vi "Read Data.vi"(8 "error in (no error)":errorcluster caption="错误输入（无错误）", 11 "Primary Productivity 输入":refnum<class "Primary Productivity.lvclass">) -> (0 "error out":errorcluster caption="错误输出", 3 "Primary Productivity 输出":refnum<class "Primary Productivity.lvclass">)   [LabVIEW 2016, in "Primary Productivity.lvclass"]
uses:
  Primary Productivity.lvclass
  Primary Productivity.lvclass/Primary Productivity.ctl
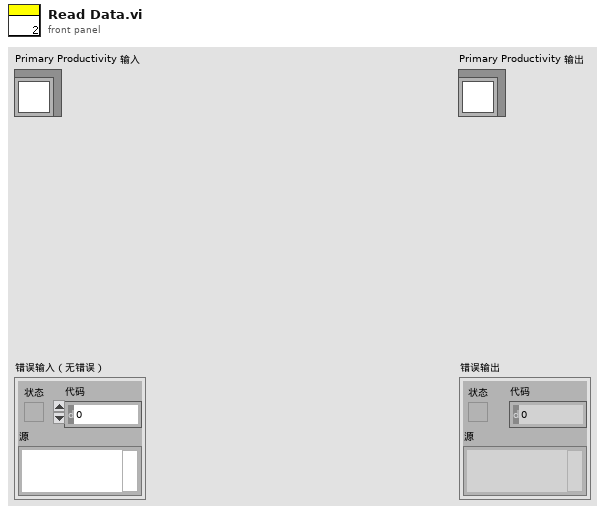
[diagram p1: front panel]
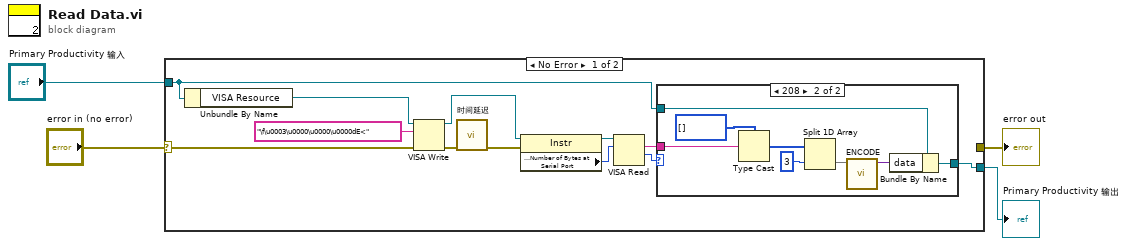
[diagram p0: block diagram]
diagram:
  n1 = case shown="No Error" "error in (no error)" {
    selector: "error in (no error)" -> [w9 w27]
    tunnel: [_ w27] -> w3
    tunnel: [w12 w26] -> w1
    tunnel: "Primary Productivity 输入" -> [w13 w26]
    frame No Error {
      n2 = Unbundle By Name(w13) -> ("VISA Resource"=w5:refnum<visa-resource-name>)
      n3 = VISA Write(VISA resource name=w5, write buffer="\f\u0003\u0000\u0000\u0000dE<" ("写入缓冲区"), error in (no error)=w9) -> (VISA resource name out=w7:refnum<visa-resource-name>, error out=w10:errorcluster)  [unwired: 1 out]
      n4 = call "时间延迟"("error in (no error)"=w10) -> ("error out"=w8:errorcluster)  [unwired: 10 in]
      n5 = property class="Instr"(reference=w7, error in=w8) -> (reference out=w16:refnum<visa-resource-name>, "Serial Settings:Number of Bytes at Serial Port"=w15:u32)  [unwired: 1 out]
      n6 = VISA Read(VISA resource name=w16, byte count=w15) -> (read buffer=w14:string, return count=w6:u32)  [unwired: 1 in, 2 out]
      n7 = case shown="208" w6 {
        tunnel: w14 -> [_ w25]
        tunnel: w13 -> [w17 w20]
        tunnel: [w17 w18] -> w12
        frame 0, Default {
        }
        frame 208 {
          n8 = Type Cast(type=u16[] [], x=w25) -> (*(type *) &x=w23:u16[])
          n9 = Split 1D Array(array=w23, index=3 ("索引")) -> (second subarray=w22:u16[])  [unwired: 1 out]
          n10 = call "ENCODE.vi"("Registers"=w22) -> ("变体"=w19:variant)  [unwired: 10 in]
          n11 = Bundle By Name(cluster=w20, "data"=w19) -> (w18:refnum<class "Primary Productivity.lvclass">)
        }
      }
    }
    frame Error {
    }
  }
  "error out" <- w3
  "Primary Productivity 输出" <- w1
